vi "_createobj4.vi"(8 "error in (no error)":errorcluster, 11 "String":string) -> (0 "error out":errorcluster, 3 "Cluster":T1)   [LabVIEW 2017]
uses:
  af16775c-c43b-4a3d-91ea-cda4722fe85e.vi
  395a29f8-5cc7-48fe-8a55-3b0722ab4507.vi
  af16775c-c43b-4a3d-91ea-cda4722fe85e.vi/2f58b0fd-b42f-49b6-a5dc-16efc1402750.vi
  395a29f8-5cc7-48fe-8a55-3b0722ab4507.vi/2f58b0fd-b42f-49b6-a5dc-16efc1402750.vi
  Data/_support/Get DataType Description String.vi
  _support/Resource.vi
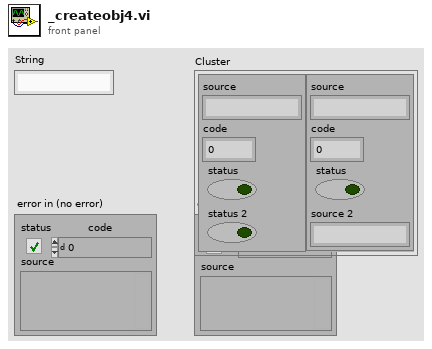
[diagram p1: front panel]
types:
  T1 = cluster{cluster{"source":string, "code":i32, "status":bool, "status 2":bool}, cluster{"source":string, "code":i32, "status":bool, "source 2":string}}
  T2 = cluster{"source":string, "code":i32, "status":bool, "source 2":string}
  T3 = cluster{"source":string, "code":i32, "status":bool, "status 2":bool}
  T4 = cluster{"Variant":cluster{"source":string, "code":i32, "status":bool, "status 2":bool}, "Variant":cluster{"source":string, "code":i32, "status":bool, "source 2":string}}
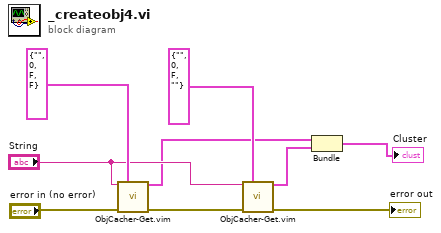
[diagram p0: block diagram]
diagram:
  n1 = call "ObjCacher-Get.vim"("Module Name"="String", "type"=T3 {"source"="", "code"=0, "status"=FALSE, "status 2"=FALSE}, "error in (no error)"="error in (no error)") -> ("Variant"=w3:T3, "error out"=w8:errorcluster)  [unwired: 9 in, 2 out]
  n2 = call "ObjCacher-Get.vim"("Module Name"="String", "type"=T2 {"source"="", "code"=0, "status"=FALSE, "source 2"=""}, "error in (no error)"=w8) -> ("Variant"=w2:T2, "error out"=→"error out":errorcluster)  [unwired: 9 in, 2 out]
  n3 = Bundle("Variant"=w3, "Variant"=w2) -> (→"Cluster":T4)  [unwired: 1 in]
